vi "Switch Debounce.vi"(10 "Time Target (s)":dbl=0.1 format="%#_13g", 11 "Switches":bool[](array[boolean])) -> (2 "Valid":bool, 3 "Debouced Switches":bool[](array[boolean]))   [LabVIEW 2017]
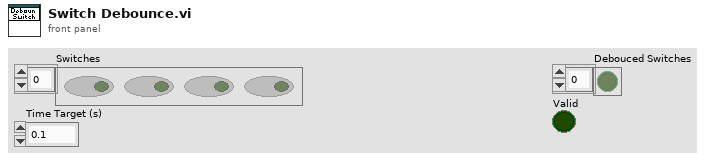
[diagram p1: front panel]
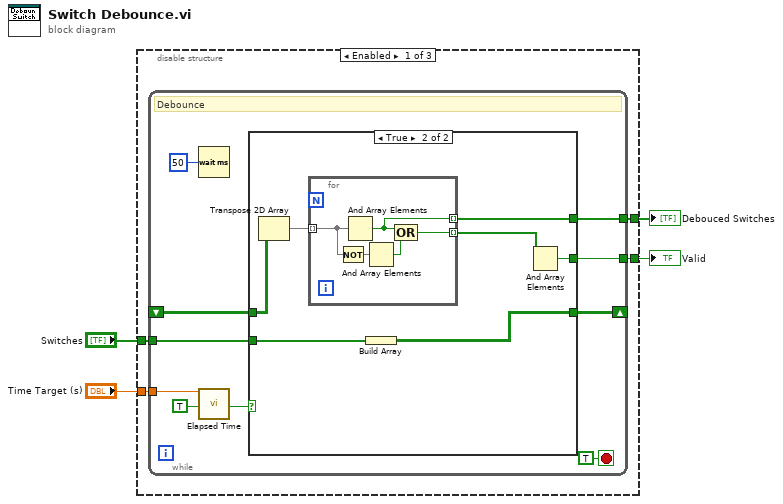
[diagram p0: block diagram]
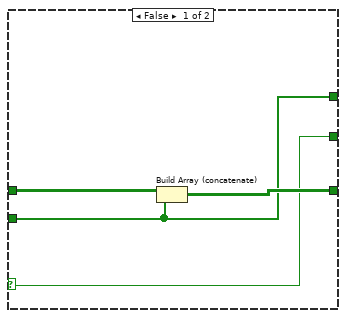
[diagram p2: hidden frame]
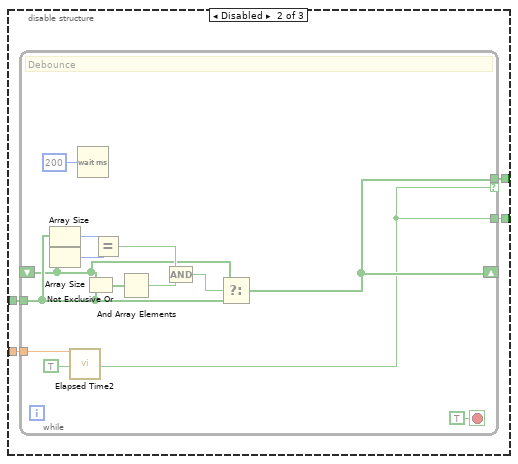
[diagram p3: hidden frame]
diagram:
  n1 = disable-structure shown="Enabled" {
    disable-tunnel: "Switches" -> [w8 w38 _]
    disable-tunnel: "Time Target (s)" -> [w7 w37 _]
    disable-tunnel: [w6 w36 _] -> w2
    disable-tunnel: [w5 w35 _] -> w1
    frame Enabled {
      n2 = while {
        tunnel: w8 -> [w14]
        tunnel: w7 -> [w17]
        shift-right: [w15] -> _
        shift-left: _ -> [w13]
        tunnel: [w11] -> w6
        tunnel: [w10] -> w5
        stop <- TRUE stop-if-true
        # "Debounce"
        n3 = Wait (ms)(milliseconds to wait=u32 50) -> ()  [unwired: 1 out]
        n4 = call "Elapsed Time"("Time Target (s)"=w17, "Auto Reset"=TRUE) -> ("Time has Elapsed"=w16:bool)  [unwired: 10 in, 7 out]
        n5 = case shown="True" w16 {
          selector: w16 -> [w19 _]
          tunnel: [w21 w28] -> w15
          tunnel: w14 -> [w20 w29]
          tunnel: w13 -> [w22 w27]
          tunnel: [w19 w23] -> w11
          tunnel: [w20 w25] -> w10
          frame False {
            n6 = Build Array (concatenate)(w22, w20) -> (w21:bool[][])
          }
          frame True {
            n7 = Transpose 2D Array(2D array=w27) -> (transposed array=w26:bool[][])
            n8 = for {
              tunnel: w26 -> [w34] mode=indexing
              tunnel: [w31] -> w25 mode=indexing
              tunnel: [w30] -> w24 mode=indexing
              n9 = Not(x=w34) -> (.not. x?=w33:bool[])
              n10 = And Array Elements(Boolean array=w34) -> (logical AND=w31:bool)
              n11 = And Array Elements(Boolean array=w33) -> (logical AND=w32:bool)
              n12 = Compound Arithmetic op=OR(w31, w32) -> (w30:bool)
            }
            n13 = Build Array(w29) -> (w28:bool[][])
            n14 = And Array Elements(Boolean array=w24) -> (logical AND=w23:bool)
          }
        }
      }
    }
    frame Disabled {
      n15 = while {
        tunnel: w38 -> [w43]
        tunnel: w37 -> [w51]
        shift-right: [w41] -> _
        shift-left: _ -> [w42]
        tunnel: [w40] -> w36
        tunnel: [w41] -> w35 if=w40
        stop <- TRUE stop-if-true
        # "Debounce"
        n16 = Array Size(array=w43) -> (size(s)=w47:i32)
        n17 = Array Size(array=w42) -> (size(s)=w46:i32)
        n18 = call "Elapsed Time2"("Time Target (s)"=w51, "Auto Reset"=TRUE) -> ("Time has Elapsed"=w40:bool)  [unwired: 10 in, 7 out]
        n19 = Wait (ms)(milliseconds to wait=u32 200) -> ()  [unwired: 1 out]
        n20 = Not Exclusive Or(1:w43, 2:w42) -> (0:w49:bool[])
        n21 = Equal?(x=w47, y=w46) -> (x = y?=w45:bool)
        n22 = And Array Elements(Boolean array=w49) -> (logical AND=w48:bool)
        n23 = Compound Arithmetic op=AND(w45, w48) -> (w44:bool)
        n24 = Select(t=w42, s=w44, f=w43) -> (s? t:f=w41:bool[])
      }
    }
    frame Disabled {
    }
  }
  "Debouced Switches" <- w1
  "Valid" <- w2
